vi "IPDialog.vi"() -> (1 "port":u16, 2 "IP":string, 3 "Cancelled?":bool)   [LabVIEW 2020]
doc: "Use this template to create a dialog box with event handling."
uses:
  global/SettingVariable.vi
  <vilib>/Utility/config.llb/Write Key (String).vi
  <vilib>/Utility/config.llb/Write Key (U32).vi
  <vilib>/Utility/config.llb/NI_LVConfig.lvlib
panel:
  in  "IP_input":string caption="IP地址："
  in  "port_input":u16 caption="端口号："
  in  "Cancel":bool
  in  "OK":bool
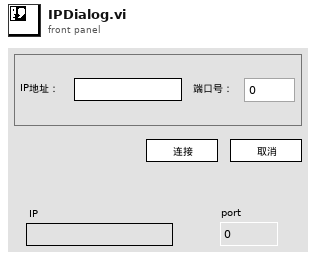
[diagram p1: front panel]
types:
  T1 = typedef "NI_LVConfig.lvlib/Config Data RefNum.ctl" = refnum<k1>
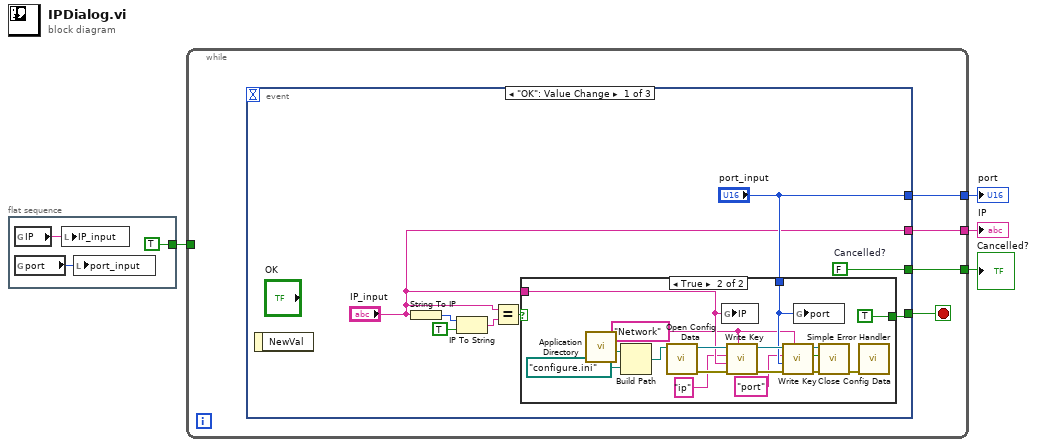
[diagram p0: block diagram]
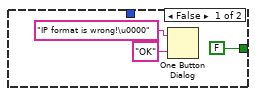
[diagram p2: hidden frame]
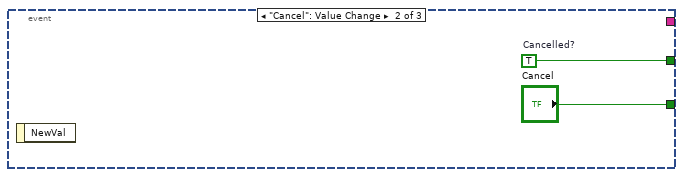
[diagram p3: hidden frame]
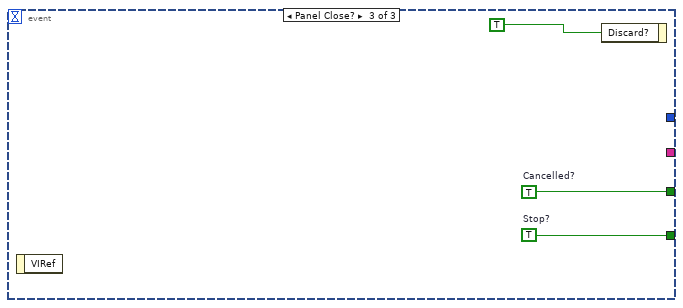
[diagram p4: hidden frame]
diagram:
  n1 = flat-sequence {
    tunnel: [TRUE] -> w1
    frame #0 {
      n2 = global read "SettingVariable.vi" "IP"() -> (w7:string)
      n3 = global read "SettingVariable.vi" "port"() -> (w6:u16)
      n4 = local write "IP_input"(w7) -> ()
      n5 = local write "port_input"(w6) -> ()
    }
  }
  n6 = while {
    tunnel: [w10] -> w4
    tunnel: [w9] -> w3
    tunnel: [w8] -> w2
    tunnel: w1 -> [_]
    stop <- w11 stop-if-true
    n7 = event shown="[0] \"OK\": Value Change" {
      selector: _ -> [_ _ _]
      dyn-events: _ -> [_ _ _]
      timeout: _ -> [_ _ _]
      tunnel: [w14 "Cancel" w43] -> w11
      tunnel: [w19 w41 w42] -> w10
      tunnel: ["IP_input" _ _] -> w9
      tunnel: ["port_input" _ _] -> w8
      event "OK": Value Change {
        w19 = FALSE  # Cancelled?
        n8 = event-data() -> ()  [unwired: 1 in, 1 out]
        n9 = String To IP(1:"IP_input") -> (0:w17:u32)
        n10 = IP To String(1:TRUE ("dot notation? (F)"), 2:w17) -> (0:w16:string)
        n11 = Equal?(x="IP_input", y=w16) -> (x = y?=w15:bool)
        n12 = case shown="True" w15 {
          tunnel: [FALSE ("Stop?") TRUE ("Stop?")] -> w14
          tunnel: "port_input" -> [_ w29]
          tunnel: "IP_input" -> [_ w30]
          frame False {
            n13 = One Button Dialog(message="IP format is wrong!\u0000", button name ("OK")="OK") -> ()  [unwired: 1 out]
          }
          frame True {
            w27 = "Network" ("section")
            n14 = call <vilib>:"Application Directory.vi"() -> ("Application Directory"=w23:path)
            n15 = Build Path(base path=w23, name or relative path=path "configure.ini") -> (appended path=w25:path)
            n16 = call <vilib>:"Open Config Data.vi"("configuration file path"=w25) -> ("error out"=w32:errorcluster, "refnum"=w33:T1)  [unwired: 2 in, 7 out]
            n17 = global write "SettingVariable.vi" "IP"(w30) -> ()
            n18 = call-poly <vilib>:"Write Key.vi"("section"=w27, "error in (no error)"=w32, "value"=w30, "key"="ip", "refnum"=w33) -> ("error out"=w38:errorcluster, "refnum out"=w37:T1)  [unwired: 4 in, 1 out]
            n19 = call-poly <vilib>:"Write Key.vi"("section"=w27, "error in (no error)"=w38, "value"=w29, "key"="port", "refnum"=w37) -> ("error out"=w36:errorcluster, "found?"=w35:bool, "refnum out"=w34:T1)  [unwired: 4 in]
            n20 = global write "SettingVariable.vi" "port"(w29) -> ()
            n21 = call <vilib>:"Close Config Data.vi"("error in (no error)"=w36, "write file if changed (T)"=w35, "refnum"=w34) -> ("error out"=w31:errorcluster)  [unwired: 8 out]
            n22 = call <vilib>:"Simple Error Handler.vi"("error in (no error)"=w31) -> ()  [unwired: 1 in, 8 out]
          }
        }
      }
      event "Cancel": Value Change {
        w41 = TRUE  # Cancelled?
        n23 = event-data() -> ()  [unwired: 1 in, 1 out]
      }
      event Panel Close? {
        w42 = TRUE  # Cancelled?
        w43 = TRUE  # Stop?
        n24 = event-data() -> ()  [unwired: 1 in, 1 out]
        n25 = event-data("Discard?"=TRUE) -> ()  [unwired: 1 in, 1 out]
      }
    }
  }
  "Cancelled?" <- w4
  "IP" <- w3
  "port" <- w2
